vi "Configure Channel (GS Sqrt).vi"(0 "VISA resource name":refnum<visa-resource-name>, 1 "Scaling":T2={"Floating point position (2)"=2, "Lower Scaling (0)"=0.0, "Upper Scaling (100.00)"=100.0, "Unit Character (\"\")"=""} {"Upper Scaling (100.00)" format="%_6g"; "Lower Scaling (0)" format="%_6g"; "Floating point position (2)" min=0 max=5 step=1}, 2 "Low cut":T1 {"Output (0: Zero)" items=["Zero", "Linear"]; "Low-cut (0)" min=0.0 max=5.0}, 5 "Channel (0001)":string="0001", 7 "Enable Channel (True)":bool=TRUE, 9 "Range, Span, Bias":T3={"GS Range (0 : 1-5V)"=0, "Enable Span (False)"=FALSE, "Lower Span (1.0000)"=1.0, "Upper Span (5.0000)"=5.0, "Bias (0)"=0.0} {"Bias (0)" format="%_6g"; "Upper Span (5.0000)" min=-99999.0 max=99999.0 step=1.0 format="%_5g"; "Lower Span (1.0000)" min=-99999.0 max=99999.0 step=1.0 format="%_5g"; "GS Range (0 : 1-5V)" items=["1-5V", "0.4-2V"]}, 11 "error in (no error)":errorcluster) -> (4 "VISA resource name out":refnum<visa-resource-name>, 6 "Channel":string, 15 "error out":errorcluster)   [LabVIEW 2020, in "Yokogawa GX Series.lvlib"]
doc: "Sets the input range as GS.\n\nCommand: SRangeAI"
uses:
  <instrlib>/Yokogawa GX Series/Yokogawa GX Series.lvlib
  <instrlib>/Yokogawa GX Series/Private/GS Range.vi
panel:
  # "%"
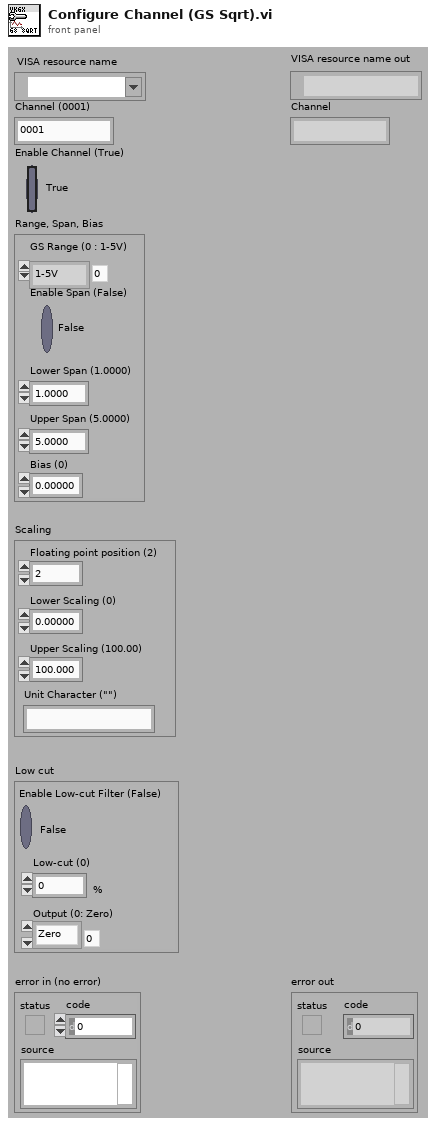
[diagram p1: front panel]
types:
  T1 = cluster{"Enable Low-cut Filter (False)":bool, "Low-cut (0)":dbl, "Output (0: Zero)":u16}
  T2 = cluster{"Floating point position (2)":i32, "Lower Scaling (0)":dbl, "Upper Scaling (100.00)":dbl, "Unit Character (\"\")":string}
  T3 = cluster{"GS Range (0 : 1-5V)":i32, "Enable Span (False)":bool, "Lower Span (1.0000)":dbl, "Upper Span (5.0000)":dbl, "Bias (0)":dbl}
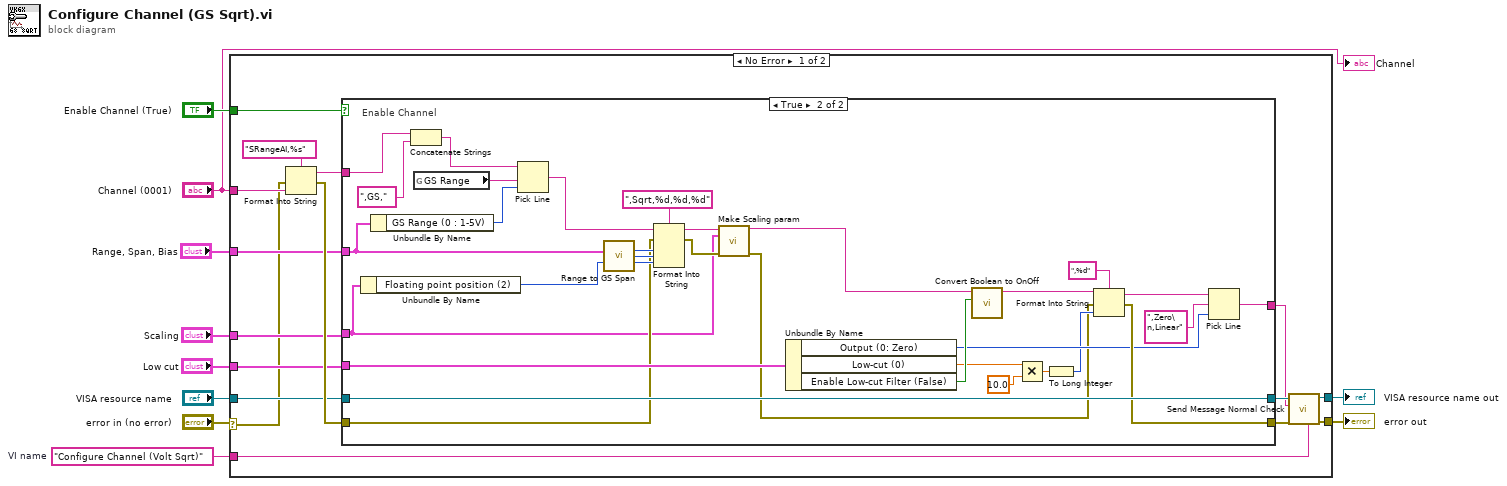
[diagram p0: block diagram]
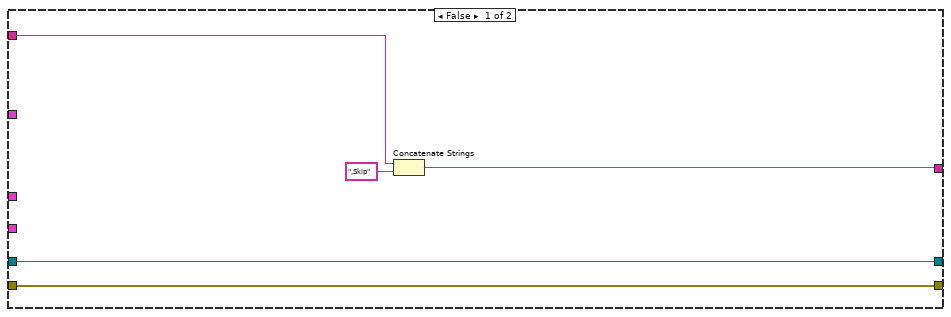
[diagram p2: hidden frame]
diagram:
  w3 = "Configure Channel (Volt Sqrt)"  # VI name
  n1 = case shown="No Error" "error in (no error)" {
    selector: "error in (no error)" -> [w11 w64]
    tunnel: "Enable Channel (True)" -> [w23 _]
    tunnel: "VISA resource name" -> [w22 w65]
    tunnel: "Range, Span, Bias" -> [w21 _]
    tunnel: "Scaling" -> [w20 _]
    tunnel: "Low cut" -> [w19 _]
    tunnel: [w16 w65] -> w5
    tunnel: [w15 w64] -> w4
    tunnel: w3 -> [w13 _]
    tunnel: "Channel (0001)" -> [w12 _]
    frame No Error {
      n2 = Format Into String(format string="SRangeAI,%s", error in=w11, w12) -> (resulting string=w24:string, error out=w25:errorcluster)  [unwired: 1 in]
      n3 = case shown="True" w23 {
        tunnel: w25 -> [w28 w45]
        tunnel: [w28 w53] -> w17
        tunnel: w24 -> [w29 w61]
        tunnel: [w31 w47] -> w14
        tunnel: w22 -> [w27 w54]
        tunnel: [w27 w54] -> w18
        tunnel: w21 -> [_ w44]
        tunnel: w20 -> [_ w36]
        tunnel: w19 -> [_ w55]
        frame False {
          n4 = Concatenate Strings(w29, ",Skip") -> (w31:string)
        }
        frame True {
          # "Enable Channel"
          n5 = Unbundle By Name(w36) -> ("Floating point position (2)"=w39:i32)
          n6 = Unbundle By Name(w44) -> ("GS Range (0 : 1-5V)"=w59:i32)
          n7 = Concatenate Strings(w61, ",GS,") -> (w60:string)
          n8 = global read "GS Range.vi" "GS Range"() -> (w32:string)
          n9 = Pick Line(string ("")=w60, multi-line string=w32, line index=w59) -> (output string=w62:string)
          n10 = call <instrlib>:"Range to GS Span.vi"("Range and span"=w44, "Floating Point Position (2)"=w39) -> ("Lower Span"=w58:i32, "Upper Span"=w57:i32, "Bias"=w56:i32)  [unwired: 11 in]
          n11 = Format Into String(format string=",Sqrt,%d,%d,%d", initial string=w62, error in=w45, w58, w57, w56) -> (resulting string=w38:string, error out=w37:errorcluster)
          n12 = call <instrlib>:"Make Scaling param.vi"("String (\"\")"=w38, "Scaling"=w36, "error in (no error)"=w37) -> ("String After"=w35:string, "error out"=w34:errorcluster)  [unwired: 11 in]
          n13 = Unbundle By Name(w55) -> ("Output (0: Zero)"=w46:u16, "Low-cut (0)"=w42:dbl, "Enable Low-cut Filter (False)"=w51:bool)
          n14 = call <instrlib>:"Convert Boolean to OnOff.vi"("On/Off"=w51, "Initial String (\"\")"=w35) -> ("Resulting String"=w49:string)  [unwired: 9 in]
          n15 = Multiply(x=w42, y=10.0) -> (x*y=w41:dbl)
          n16 = To Long Integer(number=w41) -> (32bit integer=w40:i32)
          n17 = Format Into String(format string=",%d", initial string=w49, error in=w34, w40) -> (resulting string=w48:string, error out=w53:errorcluster)
          n18 = Pick Line(string ("")=w48, multi-line string=",Zero\n,Linear", line index=w46) -> (output string=w47:string)
        }
      }
      n19 = call <instrlib>:"Send Message Normal Check.vi"("Source (\"\")"=w13, "error in (no error)"=w17, "Send Message (\"\")"=w14, "VISA resource name"=w18) -> ("error out"=w15:errorcluster, "VISA resource name out"=w16:refnum<visa-resource-name>)  [unwired: 2 in, 4 out]
    }
    frame Error {
    }
  }
  "error out" <- w4
  "VISA resource name out" <- w5
  "Channel" <- "Channel (0001)"
